vi "Read datatype.vi"(8 "error in (no error)":errorcluster, 11 "TranscriptorBasicObject in":refnum<class "TranscriptorBasicObject.lvclass">) -> (0 "error out":errorcluster, 2 "datatype":string="String*", 3 "TranscriptorBasicObject out":refnum<class "TranscriptorBasicObject.lvclass">)   [LabVIEW 2014, in "TranscriptorBasicObject.lvclass"]
uses:
  TranscriptorBasicObject.lvclass
  TranscriptorBasicObject.lvclass/TranscriptorBasicObject.ctl
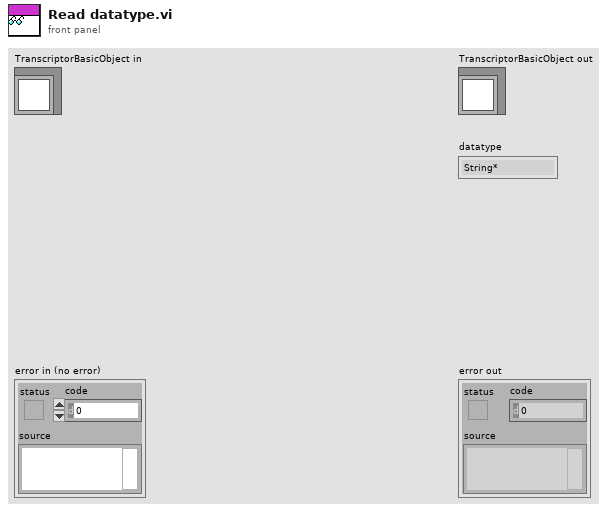
[diagram p1: front panel]
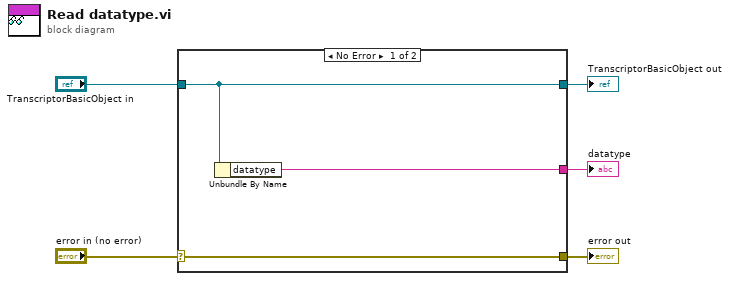
[diagram p0: block diagram]
diagram:
  n1 = case shown="No Error" "error in (no error)" {
    selector: "error in (no error)" -> [w8 w9]
    tunnel: [w8 w9] -> w4
    tunnel: [w7 w10] -> w2
    tunnel: "TranscriptorBasicObject in" -> [w7 w10]
    tunnel: [w6 _] -> w1
    frame No Error {
      n2 = Unbundle By Name(w7) -> ("datatype"=w6:string)
    }
    frame Error {
    }
  }
  "error out" <- w4
  "TranscriptorBasicObject out" <- w2
  "datatype" <- w1
